vi "Set_IO_LED_Color.vi"(8 "error in (no error)":errorcluster, 10 "SelectType":enum16{"Input", "Output"}(ring), 11 "ListBox Ref":refnum<vi>) -> (0 "error out":errorcluster)   [LabVIEW 2014]
uses:
  <vilib>/picture/picture.llb/imagedata.ctl
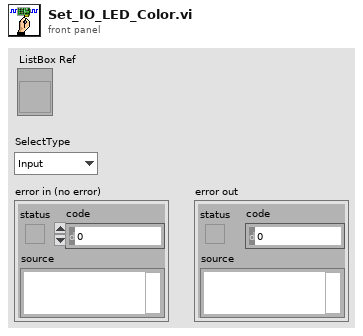
[diagram p1: front panel]
types:
  T1 = typedef "imagedata.ctl" = cluster{"image type":i32, "image depth":i32, "image":u8[], "mask":u8[], "colors":u32[], "Rectangle":cluster{"left":i16, "top":i16, "right":i16, "bottom":i16}}
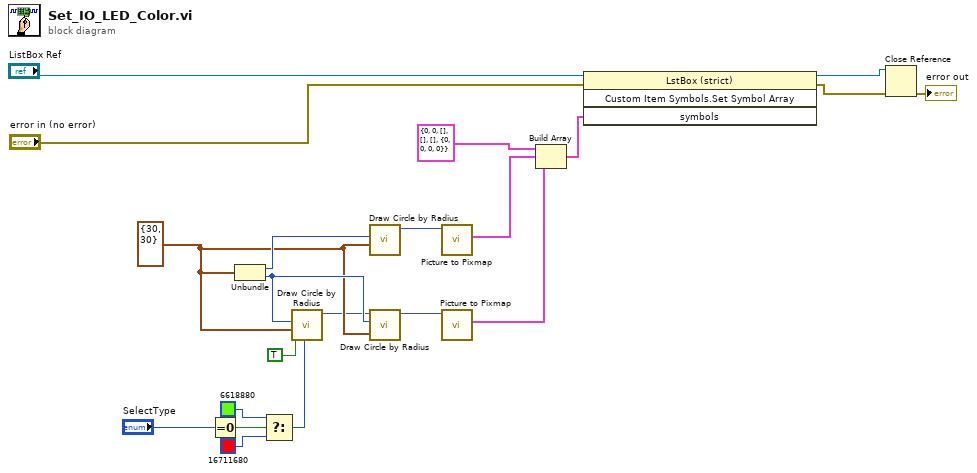
[diagram p0: block diagram]
diagram:
  w13 = cluster{"horizontal":i16, "vertical":i16} {"horizontal"=30, "vertical"=30} ("pixel center")
  n1 = Equal To 0?(x="SelectType") -> (x = 0?=w5:bool)
  n2 = Unbundle(w13) -> ("horizontal"=w14:i16, "vertical"=w15:i16)
  n3 = Select(t=u32 6618880 ("color(black)"), s=w5, f=u32 16711680 ("color(black)")) -> (s? t:f=w1:u32)
  n4 = call <vilib>:"Draw Circle by Radius.vi"("color(black)"=w1, "fill?(F)"=TRUE, "pixel center"=w13, "radius"=w15) -> ("new picture"=w11:picture)  [unwired: 7 in]
  n5 = call <vilib>:"Draw Circle by Radius.vi"("pixel center"=w13, "radius"=w14) -> ("new picture"=w10:picture)  [unwired: 9 in]
  n6 = call <vilib>:"Draw Circle by Radius.vi"("pixel center"=w13, "radius"=w15, "picture"=w11) -> ("new picture"=w12:picture)  [unwired: 8 in]
  n7 = call <vilib>:"Picture to Pixmap.vi"("picture"=w10) -> ("image data"=w8:T1)  [unwired: 9 in, 1 out]
  n8 = call <vilib>:"Picture to Pixmap.vi"("picture"=w12) -> ("image data"=w7:T1)  [unwired: 9 in, 1 out]
  n9 = Build Array(T1 {"image type"=0, "image depth"=0, "image"=[], "mask"=[], "colors"=[], "Rectangle"={"left"=0, "top"=0, "right"=0, "bottom"=0}} ("element"), w8, w7) -> (w17:T1[])
  n10 = invoke class="LstBox (strict)" method="Custom Item Symbols.Set Symbol Array"(reference="ListBox Ref", error in="error in (no error)", "symbols"=w17) -> (reference out=w19:refnum<vi>, error out=w20:errorcluster)  [unwired: 1 in, 2 out]
  n11 = Close Reference(reference=w19, error in (no error)=w20) -> (error out=→"error out":errorcluster)
